vi "Get Analog Setpoint.vi"(8 "error in (no error)":errorcluster, 11 "VISA resource name":refnum<visa-resource-name>) -> (0 "error out":errorcluster, 1 "Analog Setpoint (out)":dbl, 3 "VISA resource name out":refnum<visa-resource-name>)   [LabVIEW 2015, in "JULABO DeviceDriver.lvlib"]
doc: "This VI returns the actual setpoint adjusted via the analog interface EPROG\n\nPlease set the EPROG meaning to <B>SETPOINT</B>. See operating manual.\n\nNote:\nThis function is not available for all instruments. See operating manual to check whether your instrument supports this feature."
uses:
  JULABO DeviceDriver.lvlib
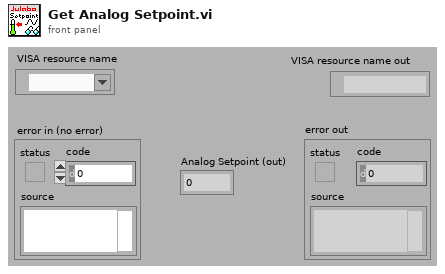
[diagram p1: front panel]
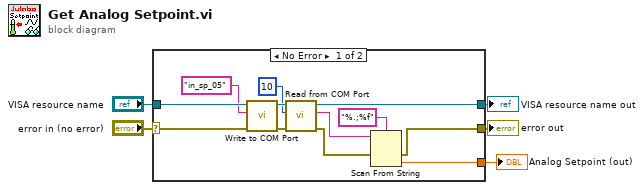
[diagram p0: block diagram]
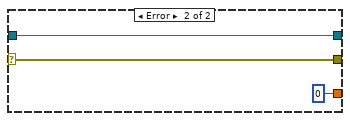
[diagram p2: hidden frame]
diagram:
  n1 = case shown="No Error" "error in (no error)" {
    selector: "error in (no error)" -> [w16 w19]
    tunnel: "VISA resource name" -> [w17 w20]
    tunnel: [w10 w19] -> w3
    tunnel: [w9 w20] -> w2
    tunnel: [w6 0] -> w1
    frame No Error {
      n2 = call "Write to COM Port.vi"("error in"=w16, "Command (input)"="in_sp_05", "VISA resource name in"=w17) -> ("error out"=w15:errorcluster, "VISA resource name out"=w14:refnum<visa-resource-name>)  [unwired: 7 in]
      n3 = call "Read from COM Port.vi"("error in"=w15, "Byte to Read (-1:All)"=u32 10 ("Anzahl der Byte"), "VISA resource name in"=w14) -> ("error out"=w12:errorcluster, "String (output)"=w11:string, "VISA resource name out"=w9:refnum<visa-resource-name>)  [unwired: 5 in, 1 out]
      n4 = Scan From String(format string="%.;%f" ("Format-String"), input string=w11, error in=w12) -> (error out=w10:errorcluster, output 1=w6:dbl)  [unwired: 2 in, 2 out]
    }
    frame Error {
    }
  }
  "error out" <- w3
  "VISA resource name out" <- w2
  "Analog Setpoint (out)" <- w1
